vi "GetOverCurrProtLimit.vi"(3 "error in (no error)":errorcluster, 5 "VISA resource name":refnum<visa-resource-name>) -> (0 "error out":errorcluster, 1 "Current":dbl, 2 "VISA resource name out":refnum<visa-resource-name>)   [LabVIEW 2019, in "9103Series.lvlib"]
uses:
  <instrlib>/9103series/9103Series.lvlib
panel:
  out "ok?":string
  out "Raw Data":string
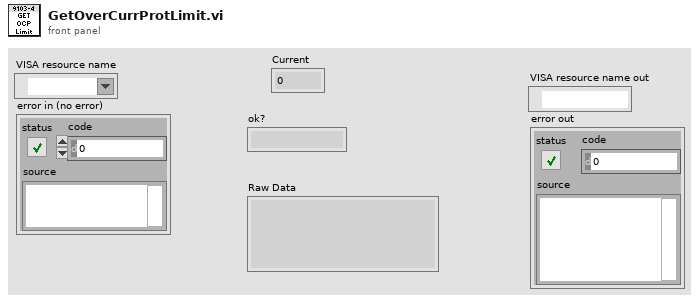
[diagram p1: front panel]
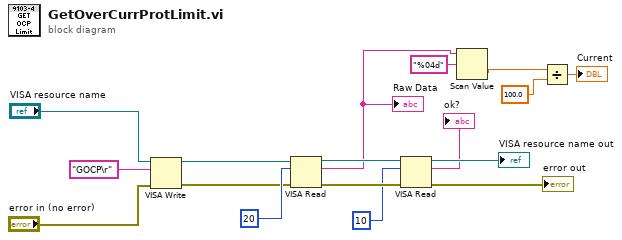
[diagram p0: block diagram]
diagram:
  n1 = VISA Write(VISA resource name="VISA resource name", write buffer="GOCP\r", error in (no error)="error in (no error)") -> (VISA resource name out=w13:refnum<visa-resource-name>, error out=w12:errorcluster)  [unwired: 1 out]
  n2 = VISA Read(VISA resource name=w13, byte count=u32 20, error in (no error)=w12) -> (VISA resource name out=w11:refnum<visa-resource-name>, read buffer=w4:string, error out=w10:errorcluster)  [unwired: 1 out]
  "Raw Data" <- w4
  n3 = VISA Read(VISA resource name=w11, byte count=u32 10, error in (no error)=w10) -> (VISA resource name out=→"VISA resource name out":refnum<visa-resource-name>, read buffer=→"ok?":string, error out=→"error out":errorcluster)  [unwired: 1 out]
  n4 = Scan Value(string=w4, format string="%04d") -> (value=w2:dbl)  [unwired: 1 in, 1 out]
  n5 = Divide(x=w2, y=100.0) -> (x/y=→"Current":dbl)
